vi "Configure Serial Bus (Flexray - Trigger - Frame).vi"(0 "VISA resource name":refnum<visa-resource-name>="MSOX3054", 1 "Frame Cycle Count Repetition (0:All)":i32(ring) items=["All", "2", "4", "8", "16", "32", "64"], 3 "Frame ID (0)":i32, 5 "Serial Bus Name (1: Serial Bus 1)":i32(ring)=1 items=["Serial Bus 1"=1, "Serial Bus 2"=2], 9 "Frame Type (7: All)":i32(ring)=7 items=["Norm", "Startup", "Null", "Sync", "NStartup", "NNull", "NSync", "All"], 11 "error in (no error)":errorcluster, 12 "Frame Cycle Count Base (-1)":i32=-1) -> (4 "VISA resource name out":refnum<visa-resource-name>="MSOX3054", 15 "error out":errorcluster)   [LabVIEW 2017, in "Agilent 2000 3000 X-Series.lvlib"]
doc: "Configures the Frame Trigger settings of FlexRay bus. The event setting is only valid when the FlexRay trigger mode is set to Frame.\n\nNote:\nThis VI is not supported by EDUX1052A/G, DSOX1202A/G, DSOX1204A/G models"
uses:
  Agilent 2000 3000 X-Series.lvlib
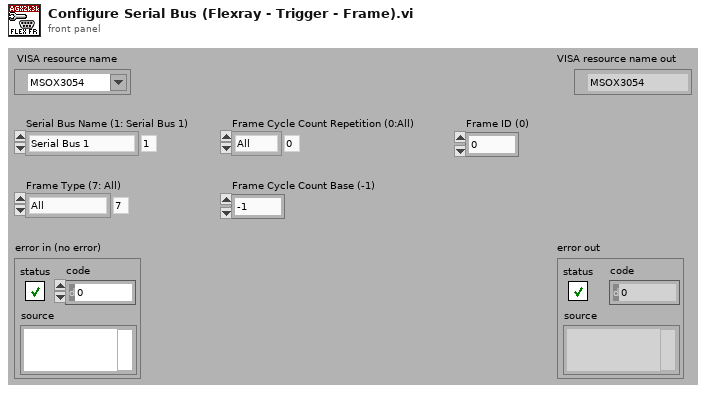
[diagram p1: front panel]
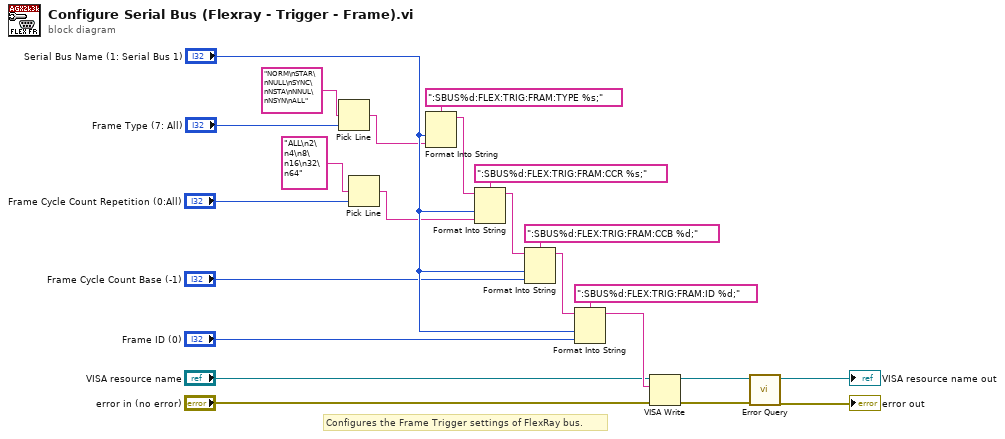
[diagram p0: block diagram]
diagram:
  # "Configures the Frame Trigger settings of FlexRay bus."
  n1 = Pick Line(multi-line string="NORM\nSTAR\nNULL\nSYNC\nNSTA\nNNUL\nNSYN\nALL", line index="Frame Type (7: All)") -> (output string=w19:string)  [unwired: 1 out]
  n2 = Pick Line(multi-line string="ALL\n2\n4\n8\n16\n32\n64", line index="Frame Cycle Count Repetition (0:All)") -> (output string=w14:string)  [unwired: 1 out]
  n3 = Format Into String(format string=":SBUS%d:FLEX:TRIG:FRAM:TYPE %s;", "Serial Bus Name (1: Serial Bus 1)", w19) -> (resulting string=w16:string)  [unwired: 2 in, 1 out]
  n4 = Format Into String(format string=":SBUS%d:FLEX:TRIG:FRAM:CCR %s;", initial string=w16, "Serial Bus Name (1: Serial Bus 1)", w14) -> (resulting string=w13:string)  [unwired: 1 in, 1 out]
  n5 = Format Into String(format string=":SBUS%d:FLEX:TRIG:FRAM:CCB %d;", initial string=w13, "Serial Bus Name (1: Serial Bus 1)", "Frame Cycle Count Base (-1)") -> (resulting string=w10:string)  [unwired: 1 in, 1 out]
  n6 = Format Into String(format string=":SBUS%d:FLEX:TRIG:FRAM:ID %d;", initial string=w10, "Serial Bus Name (1: Serial Bus 1)", "Frame ID (0)") -> (resulting string=w7:string)  [unwired: 1 in, 1 out]
  n7 = VISA Write(VISA resource name="VISA resource name", write buffer=w7, error in (no error)="error in (no error)") -> (VISA resource name out=w4:refnum<visa-resource-name>, error out=w3:errorcluster)  [unwired: 1 out]
  n8 = call "Error Query.vi"("error in (no error)"=w3, "VISA resource name"=w4) -> ("error out"=→"error out":errorcluster, "VISA resource name out"=→"VISA resource name out":refnum<visa-resource-name>)  [unwired: 8 out]
